vi "write.vi"(8 "error in":errorcluster, 9 "timeout in ms (-1)":i32=-1, 10 "element":T1, 11 "stream publisher in":refnum<class "data bus stream subscriber.lvclass">) -> (0 "error out":errorcluster, 1 "timed out?":bool, 3 "stream publisher out":refnum<class "data bus stream subscriber.lvclass">)   [LabVIEW 2013, in "data bus stream subscriber.lvclass"]
uses:
  data bus stream subscriber.lvclass
  data stream definition.ctl
  data stream message type.ctl
  data bus stream subscriber.lvclass/data bus stream subscriber.ctl
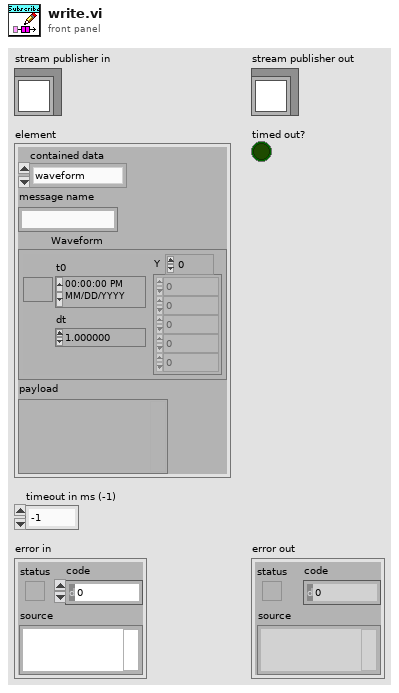
[diagram p1: front panel]
types:
  T1 = typedef "data stream definition.ctl" = cluster{"contained data":T2, "message name":string, "Waveform":waveform(dbl), "payload":variant}
  T2 = typedef "data stream message type.ctl" = enum16{"waveform", "message"}
  T3 = typedef "data bus stream subscriber.lvclass/enqueue mode.ctl" = enum16{"lossy", "lossless"}
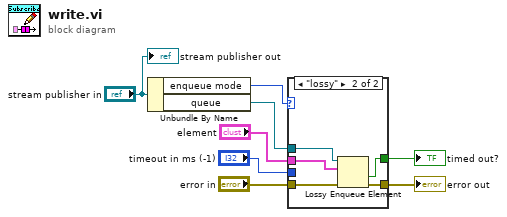
[diagram p0: block diagram]
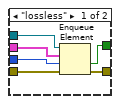
[diagram p2: hidden frame]
diagram:
  n1 = Unbundle By Name("stream publisher in") -> ("enqueue mode"=w1:T3, "queue"=w5:refnum<queue>)
  n2 = case shown="\"lossy\"" w1 {
    tunnel: "error in" -> [w14 w15]
    tunnel: [w13 w19] -> w6
    tunnel: w5 -> [w12 w18]
    tunnel: "timeout in ms (-1)" -> [w11 _]
    tunnel: [w10 w17] -> w3
    tunnel: "element" -> [w9 w16]
    frame "lossless" {
      n3 = Enqueue Element(queue=w12, element=w9, timeout in ms (-1)=w11, error in (no error)=w14) -> (timed out?=w10:bool, error out=w13:errorcluster)  [unwired: 1 out]
    }
    frame "lossy" {
      n4 = Lossy Enqueue Element(queue=w18, element=w16, error in (no error)=w15) -> (overflow?=w17:bool, error out=w19:errorcluster)  [unwired: 2 out]
    }
  }
  "error out" <- w6
  "timed out?" <- w3
  "stream publisher out" <- "stream publisher in"
